vi "Check_pipe_values.vi"(8 "error in (no error)":errorcluster, 10 "New Y-value in":dbl, 11 "Y-values":dbl[](array[numeric])) -> (0 "error out":errorcluster, 3 "New Y-value out":dbl)   [LabVIEW 2017]
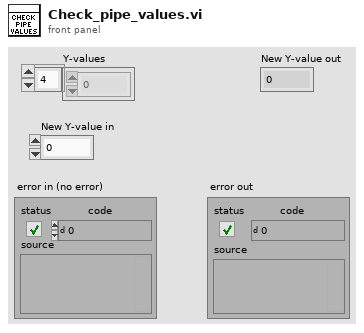
[diagram p1: front panel]
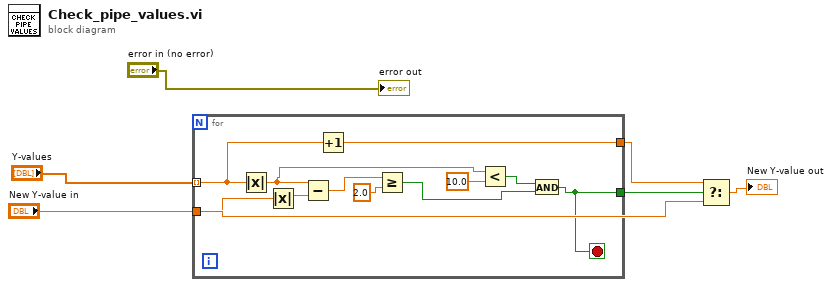
[diagram p0: block diagram]
diagram:
  n1 = for {
    tunnel: [w8] -> w6
    tunnel: "New Y-value in" -> [w13]
    tunnel: [w12] -> w3
    tunnel: "Y-values" -> [w7] mode=indexing
    stop <- w8 stop-if-true
    n2 = Absolute Value(x=w7) -> (abs(x)=w17:dbl)
    n3 = Absolute Value(x=w13) -> (abs(x)=w9:dbl)
    n4 = Subtract(x=w17, y=w9) -> (x-y=w10:dbl)
    n5 = Increment(x=w7) -> (x+1=w12:dbl)
    n6 = Greater Or Equal?(x=w10, y=2.0) -> (x >= y?=w14:bool)
    n7 = Less?(x=w17, y=10.0) -> (x < y?=w15:bool)
    n8 = And(x=w15, y=w14) -> (x .and. y?=w8:bool)
  }
  n9 = Select(t=w3, s=w6, f="New Y-value in") -> (s? t:f=→"New Y-value out":dbl)
  "error out" <- "error in (no error)"
